vi "Untitled 1.vi"() -> ()   [LabVIEW 2020]
uses:
  D:/Project/Labview-Projects/General utility tool/Libraries/HslCommunication/_Dependenciecs/HslCommunication.dll
  _Dependenciecs/HslCommunication.dll
panel:
  out "Content 2":i32[](array[numeric])
  out "Content":bool[](array[boolean])
  out "Message":string
  out "IsSuccess 2":bool
  out "IsSuccess":bool
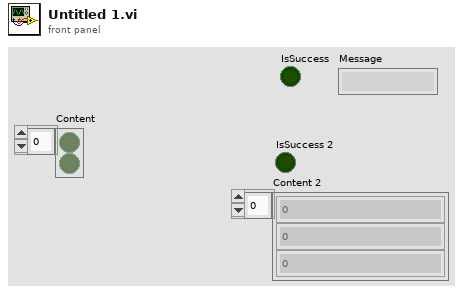
[diagram p1: front panel]
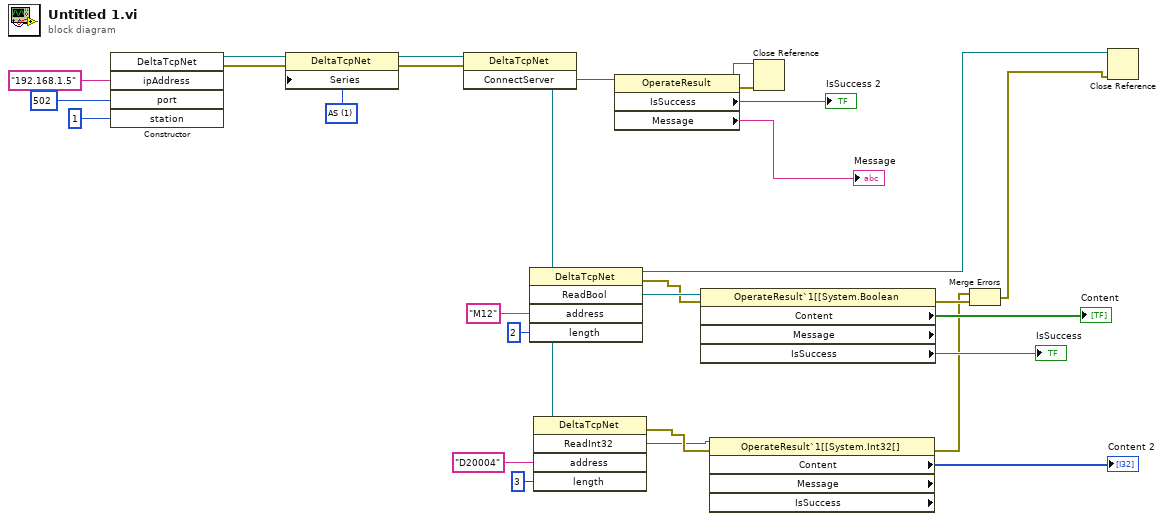
[diagram p0: block diagram]
diagram:
  w22 = 1 items=["Dvp", "AS"] ("Series")
  n1 = constructor class="DeltaTcpNet"("ipAddress"="192.168.1.5", "port"=502, "station"=u8 1) -> (reference out=w29:refnum<k24>, error out=w27:errorcluster)  [unwired: 3 in, 4 out]
  n2 = property class="DeltaTcpNet"(reference=w29, error in=w27, "Series"=w22) -> (reference out=w28:refnum<k24>, error out=w26:errorcluster)
  n3 = invoke class="DeltaTcpNet" method="ConnectServer"(reference=w28, error in=w26) -> (reference out=w1:refnum<k24>, "ConnectServer"=w21:refnum<k24>)  [unwired: 1 in, 1 out]
  n4 = invoke class="DeltaTcpNet" method="ReadBool"(reference=w1, "address"="M12", "length"=u16 2) -> (reference out=w16:refnum<k24>, error out=w15:errorcluster, "ReadBool"=w18:refnum<k24>)  [unwired: 2 in, 2 out]
  n5 = invoke class="DeltaTcpNet" method="ReadInt32"(reference=w1, "address"="D20004", "length"=u16 3) -> (error out=w6:errorcluster, "ReadInt32"=w5:refnum<k24>)  [unwired: 2 in, 3 out]
  n6 = property class="OperateResult"(reference=w21) -> (reference out=w19:refnum<k24>, error out=w20:errorcluster, "IsSuccess"=→"IsSuccess 2":bool, "Message"=→"Message":string)  [unwired: 1 in]
  n7 = property class="OperateResult`1[[System.Boolean" props=["Content", "Message", "IsSuccess"](reference=w18, error in=w15) -> (error out=w14:errorcluster, "Content"=→"Content":bool[], "IsSuccess"=→"IsSuccess":bool)  [unwired: 2 out]
  n8 = property class="OperateResult`1[[System.Int32[]" props=["Content", "Message", "IsSuccess"](reference=w5, error in=w6) -> (error out=w2:errorcluster, "Content"=→"Content 2":i32[])  [unwired: 3 out]
  n9 = Close Reference(reference=w19, error in (no error)=w20) -> ()  [unwired: 1 out]
  n10 = Merge Errors(w2, w14) -> (w3:errorcluster)
  n11 = Close Reference(reference=w16, error in (no error)=w3) -> ()  [unwired: 1 out]
